vi "MGCC_comm_global.vi"() -> ()   [LabVIEW 2016]
panel:
  out "Relay":bool[](array[boolean])
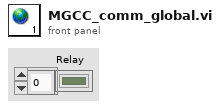
[diagram p1: front panel]
diagram:
